vi "Lightning Teleop.vi"() -> ()   [LabVIEW 2015]
uses:
  Support/Global Objects.vi
panel:
  out "error out 2":errorcluster
  in  "error in 2":errorcluster
  out "error out":errorcluster
  in  "error in":errorcluster
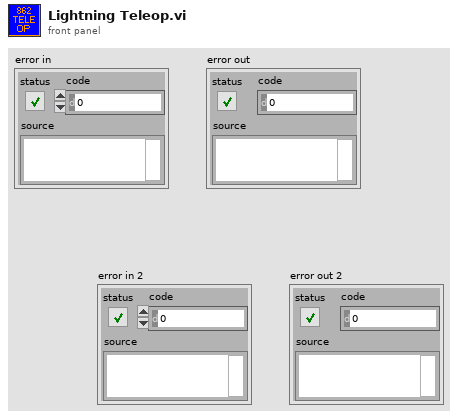
[diagram p1: front panel]
types:
  T1 = typedef "Joystick Info.ctl" = cluster{"JoystickDevRef":T2}
  T2 = typedef "WPI_JoystickDevRef.ctl" = cluster{"Device":T3}
  T3 = typedef "WPI_JoystickDeviceEnum.ctl" = enum16{"USB 0", "USB 1", "USB 2", "USB 3", "USB 4", "USB 5"}
  T4 = typedef "Teleop Commands.ctl" = cluster{"Throttle":dbl, "Turn":dbl, "Up Shift Commanded":bool, "Down Shift Commanded":bool, "Collect":bool, "Eject":bool, "Flywheel":bool, "Tank Mode":bool, "Left Motor Power":dbl, "Right Motor Power":dbl}
  T5 = typedef "Control 3.ctl" = bool[]
  T6 = typedef "Configuration.ctl" = cluster{"Throttle Dead Zone":dbl, "Throttle Ramp Rate":dbl, "Turn Dead Zone":dbl, "Auton":cluster{"Motion Plan P":dbl, "Motion Plan I":dbl, "Motion Plan D":dbl}, "Auto Upshift Enabled":bool, "Upshift Min Throttle":dbl, "Upshift Min Velocity":dbl, "Min time before upshift":dbl, "Shift Throttle Detent":u32, "Min time before downshift":dbl, "Turn PID":cluster{"Motion Plan P":dbl, "Motion Plan I":dbl, "Motion Plan D":dbl}, "Auto Coast Downshift":bool, "Downshift Coast Max Vel":dbl, "Downshift Coast Throttle Epsilon":dbl, "Left Motor Calibration":dbl, "Right Motor Calibration":dbl, "Tank Mode":bool, "Shooter PID":cluster{"Shooter  P":dbl, "Shooter  I":dbl, "Shooter  D":dbl}}
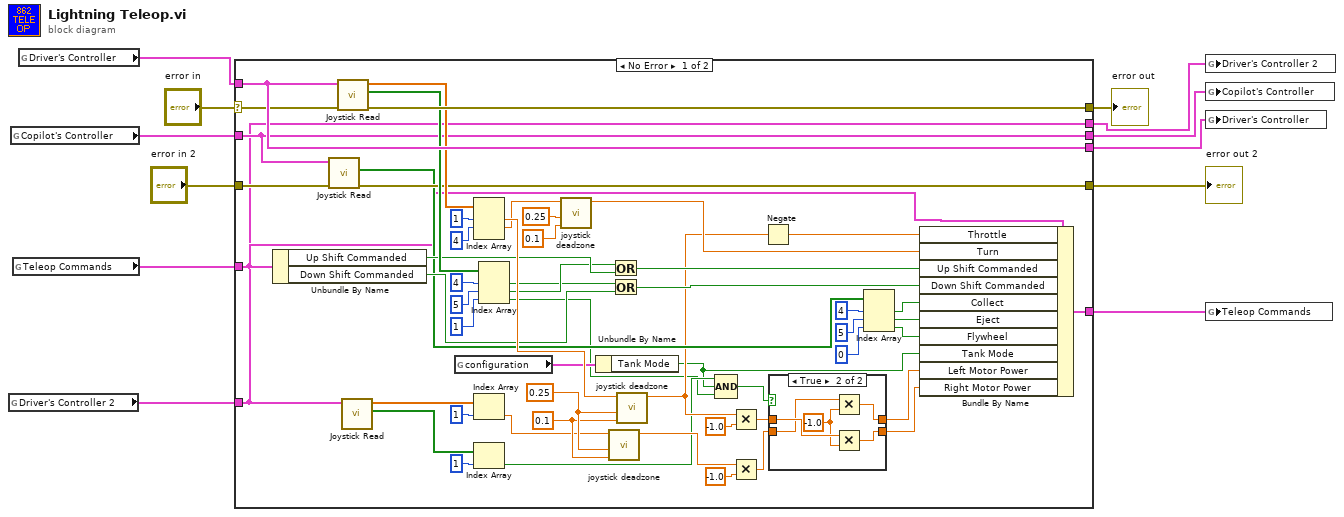
[diagram p0: block diagram]
diagram:
  n1 = global read "Global Objects.vi" "Driver's Controller 2"() -> (w2:T1)
  n2 = global read "Global Objects.vi" "Copilot's Controller"() -> (w4:T1)
  n3 = global read "Global Objects.vi" "Teleop Commands"() -> (w8:T4)
  n4 = global read "Global Objects.vi" "Driver's Controller"() -> (w10:T1)
  n5 = case shown="No Error" "error in" {
    selector: "error in" -> [w66 w80]
    tunnel: [w65 w80] -> w11
    tunnel: [w67 w79] -> w9
    tunnel: w10 -> [w67 w79]
    tunnel: w8 -> [w41 w78]
    tunnel: [w61 w78] -> w7
    tunnel: [w47 w77] -> w6
    tunnel: "error in 2" -> [w46 w77]
    tunnel: w4 -> [w45 w76]
    tunnel: [w45 w76] -> w3
    tunnel: w2 -> [w27 w75]
    tunnel: [w27 w75] -> w1
    frame No Error {
      w33 = 0.1 ("minpower")
      w34 = 0.25 ("deadzone")
      n6 = Unbundle By Name(w41) -> ("Up Shift Commanded"=w53:bool, "Down Shift Commanded"=w49:bool)
      n7 = call "Joystick Read.vi"("error in"=w46, "Joystick In"=w45) -> ("error out"=w47:errorcluster, "Buttons"=w42:T5)  [unwired: 6 in, 2 out]
      n8 = call "Joystick Read.vi"("error in"=w66, "Joystick In"=w67) -> ("error out"=w65:errorcluster, "Buttons"=w56:T5, "Axes"=w64:dbl[])  [unwired: 6 in, 1 out]
      n9 = call "Joystick Read.vi"("Joystick In"=w27) -> ("Buttons"=w23:T5, "Axes"=w26:dbl[])  [unwired: 7 in, 2 out]
      n10 = global read "Global Objects.vi" "configuration"() -> (w28:T6)
      n11 = Index Array(array=w64, index #1=1 ("index"), index #2=4 ("index")) -> (element #1=w62:dbl, element #2=w57:dbl)  [unwired: 1 in, 1 out]
      n12 = Index Array(array=w26, index=1) -> (element=w24:dbl)
      n13 = Index Array(array=w23, index=1) -> (element=w20:bool)
      n14 = Index Array(array=w56, index #1=4 ("index"), index #2=5 ("index"), index #3=1 ("index")) -> (element #1=w50:bool, element #2=w52:bool, element #3=w18:bool)
      n15 = call "joystick deadzone.vi"("minpower"=0.1, "deadzone"=0.25, "joystick"=w57) -> ("joyout"=w36:dbl)  [unwired: 8 in]
      n16 = Unbundle By Name(w28) -> ("Tank Mode"=w19:bool)
      n17 = call "joystick deadzone.vi"("minpower"=w33, "deadzone"=w34, "joystick"=w24) -> ("joyout"=w29:dbl)  [unwired: 8 in]
      n18 = Or(x=w52, y=w53) -> (x .or. y?=w51:bool)
      n19 = Or(x=w50, y=w49) -> (x .or. y?=w48:bool)
      n20 = call "joystick deadzone.vi"("minpower"=w33, "deadzone"=w34, "joystick"=w62) -> ("joyout"=w32:dbl)  [unwired: 8 in]
      n21 = Compound Arithmetic op=AND(w20, w19, w18) -> (w17:bool)
      n22 = Multiply(x=w32, y=-1.0) -> (x*y=w14:dbl)
      n23 = Multiply(x=w29, y=-1.0) -> (x*y=w16:dbl)
      n24 = Negate(x=w32) -> (-x=w35:dbl)
      n25 = case shown="True" w17 {
        tunnel: [w69 w73] -> w15
        tunnel: w16 -> [w69 w72]
        tunnel: w14 -> [w68 w74]
        tunnel: [w68 w70] -> w13
        frame False {
        }
        frame True {
          w71 = -1.0 ("y")
          n26 = Multiply(x=w72, y=w71) -> (x*y=w70:dbl)
          n27 = Multiply(x=w74, y=w71) -> (x*y=w73:dbl)
        }
      }
      n28 = Index Array(array=w42, index #1=4 ("index"), index #2=5 ("index"), index #3=0 ("index")) -> (element #1=w40:bool, element #2=w39:bool, element #3=w37:bool)
      n29 = Bundle By Name "Bundle By Name"(cluster=w41, "Throttle"=w35, "Turn"=w36, "Up Shift Commanded"=w51, "Down Shift Commanded"=w48, "Collect"=w40, "Eject"=w39, "Flywheel"=w37, "Tank Mode"=w19, "Left Motor Power"=w13, "Right Motor Power"=w15) -> (w61:T4)
    }
    frame Error {
    }
  }
  "error out" <- w11
  "error out 2" <- w6
  n30 = global write "Global Objects.vi" "Driver's Controller 2"(w1) -> ()
  n31 = global write "Global Objects.vi" "Copilot's Controller"(w3) -> ()
  n32 = global write "Global Objects.vi" "Driver's Controller"(w9) -> ()
  n33 = global write "Global Objects.vi" "Teleop Commands"(w7) -> ()
